vi "mx position control test constant.vi"() -> ()   [LabVIEW 2016]
uses:
  <instrlib>/Dynamixel Motor/Public/Motor Operation/Low Level/Baud Setting.ctl
  <vilib>/myRIO/Instrument Drivers/Onboard IO/DIO/typedefs/DIO Reference.ctl
  <vilib>/myRIO/Common/Instrument Driver Framework/Utilities/typedefs/myRIO Generic Hardware Reference.ctl
  <vilib>/myRIO/Common/Instrument Driver Framework/Utilities/typedefs/Hardware Version Enum.ctl
  <vilib>/myRIO/Common/Instrument Driver Framework/Utilities/typedefs/myRIO v1.0 Reference.ctl
  <vilib>/myRIO/Common/Instrument Driver Framework/Utilities/typedefs/Generic FPGA Reference.ctl
  <vilib>/myRIO/Common/Instrument Driver Framework/myRIO v1.0/DIO/typedefs/DIO Channels List.ctl
  <vilib>/myRIO/Common/Instrument Driver Framework/myRIO v1.0/DIO/typedefs/DIO Channels Enum.ctl
  <vilib>/userdefined/High Color/nirio_resource_hc.ctl
  <vilib>/myRIO/Common/Instrument Driver Framework/Utilities/vis/Is FPGA Ref Available.vi
  <vilib>/myRIO/Common/Instrument Driver Framework/myRIO v1.0/DIO/vis/myRIO v1.1 Open DIO.vi
  <vilib>/myRIO/Instrument Drivers/Onboard IO/DIO/vis/Write.vi
  <vilib>/myRIO/Common/Instrument Driver Framework/Utilities/vis/Validate Channels.vi
  <vilib>/myRIO/Common/Instrument Driver Framework/myRIO v1.0/DIO/vis/myRIO v1.0 Reserve DIO.vi
  <vilib>/myRIO/Common/Instrument Driver Framework/myRIO v1.0/Resource Manager/vis/myRIO v1.0 Reserve Channel List.vi
  <vilib>/myRIO/Common/Instrument Driver Framework/myRIO v1.0/DIO/vis/myRIO v1.0 Build MUX Configuration DIO.vi
  <vilib>/myRIO/Common/Instrument Driver Framework/myRIO v1.0/Resource Manager/vis/myRIO v1.0 Reserve Channel.vi
  <vilib>/myRIO/Common/Instrument Driver Framework/myRIO v1.0/Resource Manager/vis/myRIO v1.0 Unreserve Channel.vi
  <vilib>/myRIO/Common/Instrument Driver Framework/myRIO v1.0/Resource Manager/vis/myRIO v1.0 Create Configuration List.vi
  <vilib>/myRIO/Common/Instrument Driver Framework/myRIO v1.0/Resource Manager/vis/myRIO v1.0 Build Mutex Name.vi
  <vilib>/Utility/VariantDataType/GetNumericInfo.vi
  <vilib>/Utility/error.llb/Error Cluster From Error Code.vi
  <vilib>/myRIO/Common/Instrument Driver Framework/myRIO v1.0/myRIO v1.1 Open.vi
  <vilib>/myRIO/Common/Instrument Driver Framework/Utilities/vis/IO Manager.vi
  <vilib>/myRIO/Common/Instrument Driver Framework/Utilities/vis/Configuration Manager.vi
  <vilib>/myRIO/Common/Instrument Driver Framework/myRIO v1.0/Resource Manager/vis/myRIO v1.0 Configure IO.vi
  <vilib>/myRIO/Common/Instrument Driver Framework/myRIO v1.0/myRIO v1.0 Close.vi
  <vilib>/myRIO/Common/Instrument Driver Framework/myRIO v1.0/DIO/vis/myRIO v1.0 Write DIO.vi
  <vilib>/myRIO/Express VI/Onboard Devices/LED/LED Express VI.xnode
  <vilib>/myRIO/Instrument Drivers/Onboard IO/DIO/vis/myRIO DIO Open.xnode
  <instrlib>/Dynamixel Motor/Dynamixel Motor.lvlib
  <vilib>/myRIO/Instrument Drivers/Onboard IO/DIO/DIO.lvlib
panel:
  in  "Goal position":dbl
  out "Position (deg) 2":dbl
  in  "Motor ID (0)":u8=4
  in  "LED0":bool
  out "Load/torque %":sgl
  out "x+y":dbl
  out "Position (deg)":dbl
  in  "정지":bool
  # "Motor 1 Configuration"
  # "Motor 2 Configuration"
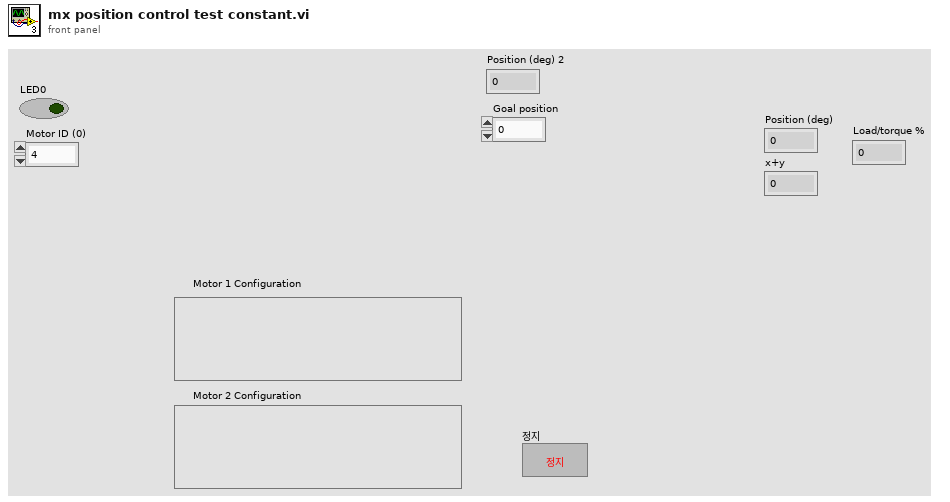
[diagram p1: front panel]
types:
  T1 = typedef "Dynamixel Motor.lvlib/Baud Setting.ctl" = u8
  T2 = typedef "DIO.lvlib/DIO Reference.ctl" = cluster{"myRIO Reference":T3, "DIO Channels List":T7}
  T3 = typedef "myRIO Generic Hardware Reference.ctl" = cluster{"myRIO Model":T4, "myRIO Hardware Reference":T5}
  T4 = typedef "Hardware Version Enum.ctl" = enum16{"Unknown", "myRIO-1900", "myRIO-1950", "roboRIO", "NI ELVIS RIO CM"}
  T5 = typedef "myRIO v1.0 Reference.ctl" = cluster{"Generic FPGA Reference":T6, "Allow multiple opens":bool}
  T6 = typedef "Generic FPGA Reference.ctl" = refnum<k20>
  T7 = typedef "DIO Channels List.ctl" = T8[]
  T8 = typedef "DIO Channels Enum.ctl" = enum16{"Not Connected", "C/DIO0", "C/DIO1", "C/DIO2", "C/DIO3", "C/DIO4", "C/DIO5", "C/DIO6", "C/DIO7", "A/DIO0", "A/DIO1", "A/DIO2", "A/DIO3", "A/DIO4", "A/DIO5", "A/DIO6", "A/DIO7", "A/DIO8", "A/DIO9", "A/DIO10", "A/DIO11", "A/DIO12", "A/DIO13", "A/DIO14", "A/DIO15", "B/DIO0", "B/DIO1", "B/DIO2", "B/DIO3", "B/DIO4", "B/DIO5", "B/DIO6", "B/DIO7", "B/DIO8", "B/DIO9", "B/DIO10", "B/DIO11", "B/DIO12", "B/DIO13", "B/DIO14", "B/DIO15", "LED0", "LED1", "LED2", "LED3", "Button0", "DIO/DIO0", "DIO/DIO1", "DIO/DIO2", "DIO/DIO3", "DIO/DIO4", "DIO/DIO5", "DIO/DIO6", "DIO/DIO7", "DIO/DIO8", "DIO/DIO9", "SPI/CS0", "SPI/CS1", "SPI/CS2", "SPI/CS3", "LED RADIO (Green)", "LED RADIO (Red)", "LED COMM (Green)", "LED COMM (Red)", "LED MODE (Green)", "LED MODE (Red)"}
  T9 = typedef "nirio_resource_hc.ctl" = tag
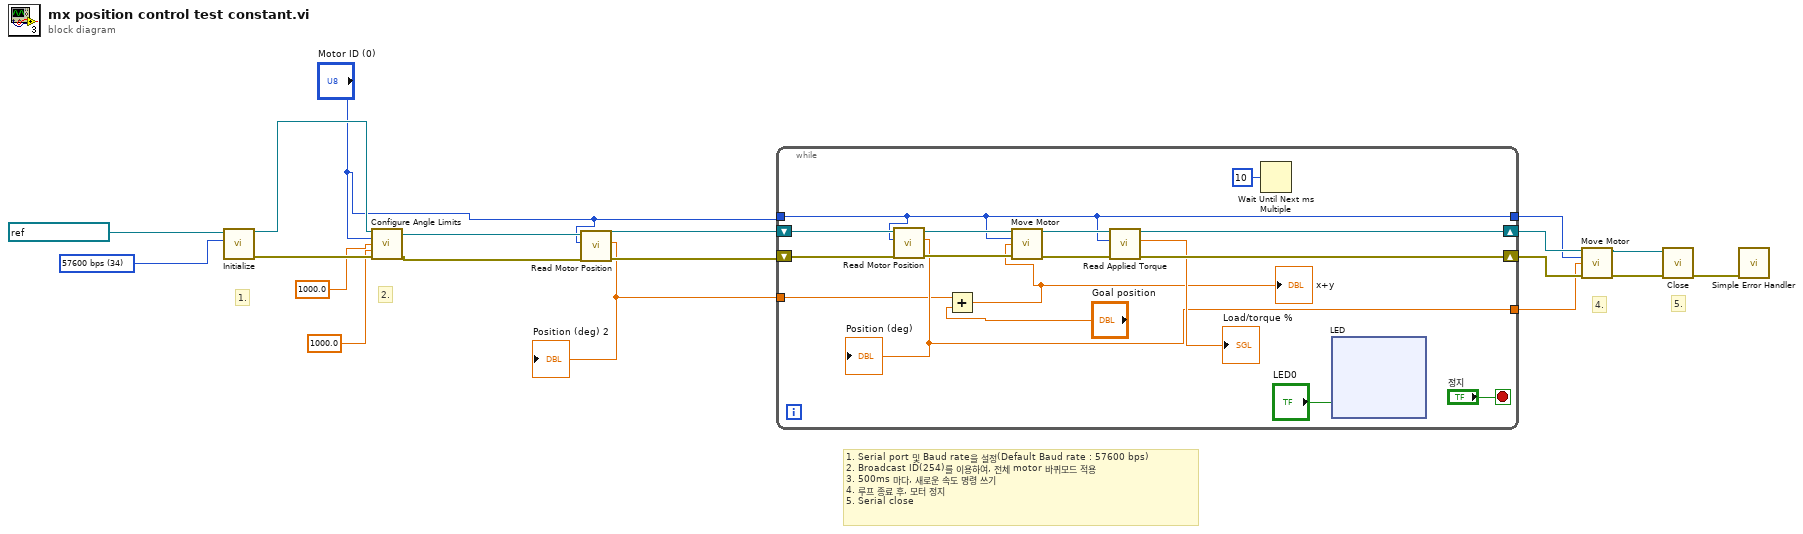
[diagram p0: block diagram]
diagram:
  w17 = T1 34 items=["1,000,000 bps"=1, "500,000 bps"=3, "400,000 bps"=4, "250,000 bps"=7, "200,000 bps"=9, "115200 bps"=16, "57600 bps"=34, "19200 bps"=103, "9600 bps"=207] ("Baud rate (57600 bps)")
  # "5."
  # "1. Serial port 및 Baud rate을 설정(Default Baud rate : 57600 bps)\n2. Broadcast ID(254)를 이용하여, 전체 motor 바퀴모드 적용\n3. 500ms 마다, 새로운 속도 명령 쓰기\n4. 루프 종료 후, 모터 정지\n5. Serial close"
  # "2."
  # "4."
  # "1."
  n1 = call <instrlib>:"Initialize.vi"("Baud rate (57600 bps)"=w17, "VISA resource name"=refnum<visa-resource-name> "ASRL3::INSTR") -> ("error out"=w19:errorcluster, "VISA resource name out"=w12:refnum<visa-resource-name>)  [unwired: 8 in]
  n2 = call <instrlib>:"Configure Angle Limits.vi"("VISA resource name"=w12, "Motor ID (0)"="Motor ID (0)", "Clockwise Angle Limit (0 deg)"=1000.0, "Counter-Clockwise Angle Limit (360 deg)"=1000.0, "error in (no error)"=w19) -> ("VISA resource name out"=w3:refnum<visa-resource-name>, "error out"=w6:errorcluster)  [unwired: 9 in]
  n3 = call <instrlib>:"Read Motor Position.vi"("error in (no error)"=w6, "Motor ID (0)"="Motor ID (0)", "VISA resource name"=w3) -> ("error out"=w5:errorcluster, "Position (deg)"=w1:dbl, "VISA resource name out"=w4:refnum<visa-resource-name>)  [unwired: 6 in]
  "Position (deg) 2" <- w1
  n4 = while {
    shift-right: [w27] -> w15
    shift-left: w4 -> [w34]
    shift-right: [w28] -> w14
    shift-left: w5 -> [w33]
    tunnel: "Motor ID (0)" -> [w26]
    tunnel: [w26] -> w9
    tunnel: [w23] -> w7
    tunnel: w1 -> [w22]
    stop <- "정지" stop-if-true
    n5 = call <instrlib>:"Read Motor Position.vi"("error in (no error)"=w33, "Motor ID (0)"=w26, "VISA resource name"=w34) -> ("error out"=w32:errorcluster, "Position (deg)"=w23:dbl, "VISA resource name out"=w31:refnum<visa-resource-name>)  [unwired: 6 in]
    "Position (deg)" <- w23
    n6 = Add(x=w22, y="Goal position") -> (x+y=w20:dbl)
    "x+y" <- w20
    n7 = call <instrlib>:"Move Motor.vi"("VISA resource name"=w31, "Motor ID (0)"=w26, "Goal Position (180 deg)"=w20, "error in (no error)"=w32) -> ("VISA resource name out"=w30:refnum<visa-resource-name>, "error out"=w29:errorcluster)  [unwired: 10 in]
    n8 = call <instrlib>:"Read Applied Torque.vi"("error in (no error)"=w29, "Motor ID (0)"=w26, "VISA resource name"=w30) -> ("error out"=w28:errorcluster, "Load/torque %"=→"Load/torque %":sgl, "VISA resource name out"=w27:refnum<visa-resource-name>)  [unwired: 6 in]
    n9 = Wait Until Next ms Multiple(millisecond multiple=u32 10 ("ms 배수")) -> ()  [unwired: 1 out]
    n10 = xnode "LED"("LED0"="LED0") -> ()  [unwired: 1 in, 1 out]
  }
  n11 = call <instrlib>:"Move Motor.vi"("VISA resource name"=w15, "Motor ID (0)"=w9, "Goal Position (180 deg)"=w7, "error in (no error)"=w14) -> ("VISA resource name out"=w13:refnum<visa-resource-name>, "error out"=w16:errorcluster)  [unwired: 10 in]
  n12 = call <instrlib>:"Close.vi"("error in (no error)"=w16, "VISA resource name"=w13) -> ("error out"=w18:errorcluster)  [unwired: 9 in]
  n13 = call <vilib>:"Simple Error Handler.vi"("error in (no error)"=w18) -> ()  [unwired: 4 in, 5 out]
